vi "lighting_property_to_opengl.vi"(2 "Lighting Properties":T2) -> (1 "Cutoff":dbl, 4 "Exponent":dbl, 5 "Ambient Color":cluster{"R":sgl, "G":sgl, "B":sgl, "A":sgl}, 6 "Diffuse Color":cluster{"R":sgl, "G":sgl, "B":sgl, "A":sgl}, 7 "Specular Color":cluster{"R":sgl, "G":sgl, "B":sgl, "A":sgl}, 8 "Attenuation":T1)   [LabVIEW 2020, in "3DPC_SurfacePlot.xctl"]
uses:
  <vilib>/Native 3D Graph/xcontrol/3DPC_SurfacePlot.xctl
  <vilib>/Native 3D Graph/typedefs/prop_lighting.ctl
  <vilib>/Utility/miscctls.llb/LVAttenuationTypeDef.ctl
  <vilib>/picture/3D Picture Control/NI_3D Picture Control.lvlib
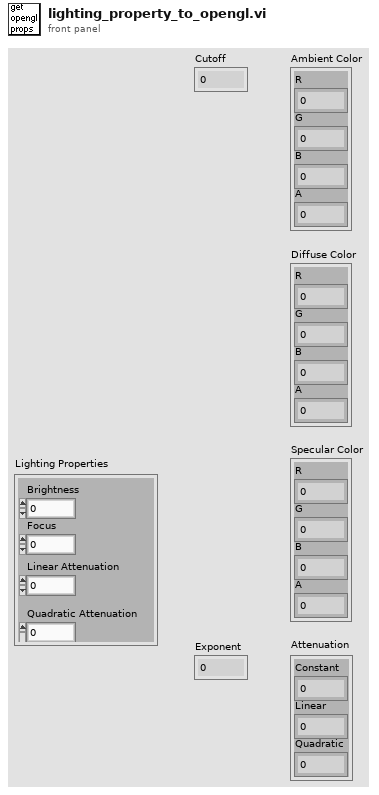
[diagram p1: front panel]
types:
  T1 = typedef "LVAttenuationTypeDef.ctl" = cluster{"Constant":sgl, "Linear":sgl, "Quadratic":sgl}
  T2 = typedef "3DPC_SurfacePlot.xctl/prop_lighting.ctl" = cluster{"Brightness":i32, "Focus":dbl, "Linear Attenuation":dbl, "Quadratic Attenuation":dbl}
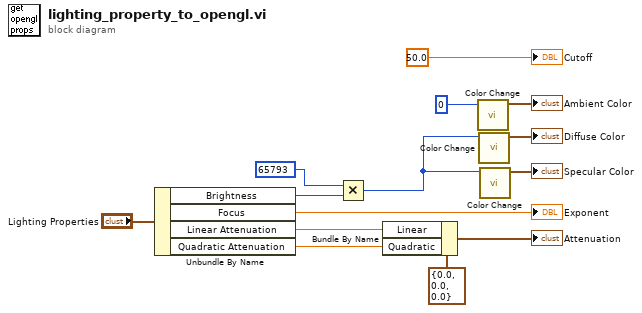
[diagram p0: block diagram]
diagram:
  n1 = Unbundle By Name("Lighting Properties") -> ("Brightness"=w13:i32, "Focus"=→"Exponent":dbl, "Linear Attenuation"=w8:dbl, "Quadratic Attenuation"=w7:dbl)
  n2 = Multiply(x=65793, y=w13) -> (x*y=w3:i32)
  n3 = Bundle By Name(cluster=T1 {"Constant"=0.0, "Linear"=0.0, "Quadratic"=0.0} ("Attenuation"), "Linear"=w8, "Quadratic"=w7) -> (→"Attenuation":T1)
  n4 = call <vilib>:"Color Change.vi"("Color"=0 ("Ambient Color")) -> ("RGBA"=→"Ambient Color":cluster{"R":sgl, "G":sgl, "B":sgl, "A":sgl})  [unwired: 1 in, 9 out]
  n5 = call <vilib>:"Color Change.vi"("Color"=w3) -> ("RGBA"=→"Diffuse Color":cluster{"R":sgl, "G":sgl, "B":sgl, "A":sgl})  [unwired: 1 in, 9 out]
  n6 = call <vilib>:"Color Change.vi"("Color"=w3) -> ("RGBA"=→"Specular Color":cluster{"R":sgl, "G":sgl, "B":sgl, "A":sgl})  [unwired: 1 in, 9 out]
  "Cutoff" <- 50.0 ("Cutoff")
